vi "RUS Sweep -- write line to log file.vi"(6 "temperature boxes":T1={"LTC21 Address"="GPIB0::15::INSTR", "ITC503 Address"="GPIB0::24::INSTR", "ITC temperature"=299.2, "ITC set temperature"=295.0, "LTC temperature"=0.0, "heater"=0.0, "gas flow"=90.0, "P"=10.0, "D"=1.0, "I"=3.0, "ITC state"="X0A1C2S00H1L0\r", "nonzero temperature"=0.0, "Magn Field (T)"=0.0, "LakeShore340"="", "LS340 Adress"=0, "Sample Temperature Source"=enum."read T <- LakeShore 340", "Neocera sensor"=1}, 7 "base path":path, 8 "error in (no error)":errorcluster, 9 "current sweep file name":string="Stability_", 10 "base name":string="Stability_", 11 "thermometer snapshot":T3={"ITC Temperature"=0.0, "ITC Set Temperature"=0.0, "LTC Temperature"=0.0, "LTC21 Address"="GPIB0::15::INSTR", "ITC503 Address"="GPIB0::24::INSTR"}) -> (0 "error out":errorcluster={"status"=TRUE, "code"=-200019, "source"="DAQmx Read (Analog 1D Wfm NChan NSamp).vi:1<append>\n<B>Task Name: </B>_unnamedTask<2C36>"}, 2 "writing to":string, 3 "log line":string="time=Jun11,2011__19:39:45\tLTC=141.78200\tITC=142.45000\t ITC_set=142.45000\t\t filename=141.78200K_300_3300_061111.dat\t")   [LabVIEW 2015]
uses:
  state.ctl
  Sample_Temperature_Source_Control.ctl
  <vilib>/Utility/file.llb/Write To Spreadsheet File (string).vi
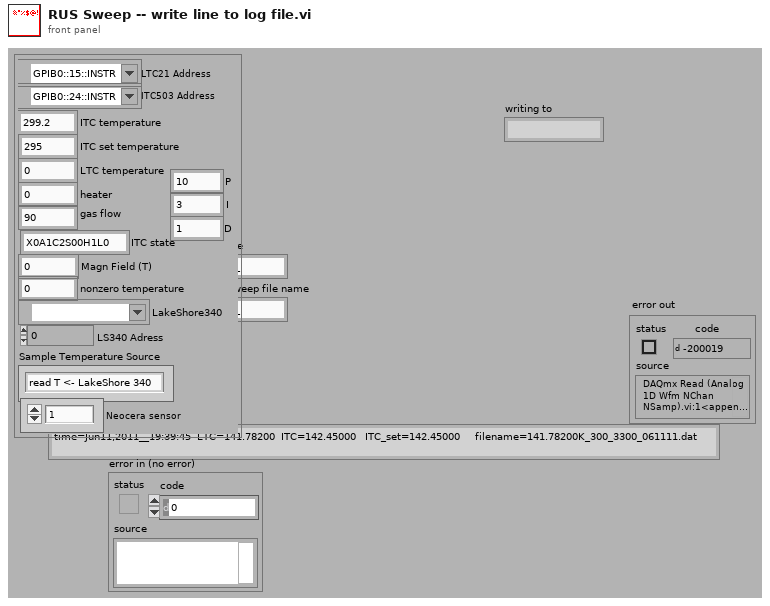
[diagram p1: front panel]
types:
  T1 = typedef "state.ctl" = cluster{"LTC21 Address":refnum<visa-resource-name>, "ITC503 Address":refnum<visa-resource-name>, "ITC temperature":dbl, "ITC set temperature":dbl, "LTC temperature":dbl, "heater":dbl, "gas flow":dbl, "P":dbl, "D":dbl, "I":dbl, "ITC state":string, "nonzero temperature":dbl, "Magn Field (T)":dbl, "LakeShore340":refnum<visa-resource-name>, "LS340 Adress":i16, "Sample Temperature Source":T2, "Neocera sensor":i32}
  T2 = typedef "Sample_Temperature_Source_Control.ctl" = enum16{"read T <- LakeShore 340", "read T <- Neocera"}
  T3 = cluster{"ITC Temperature":dbl, "ITC Set Temperature":dbl, "LTC Temperature":dbl, "LTC21 Address":refnum<visa-resource-name>, "ITC503 Address":refnum<visa-resource-name>}
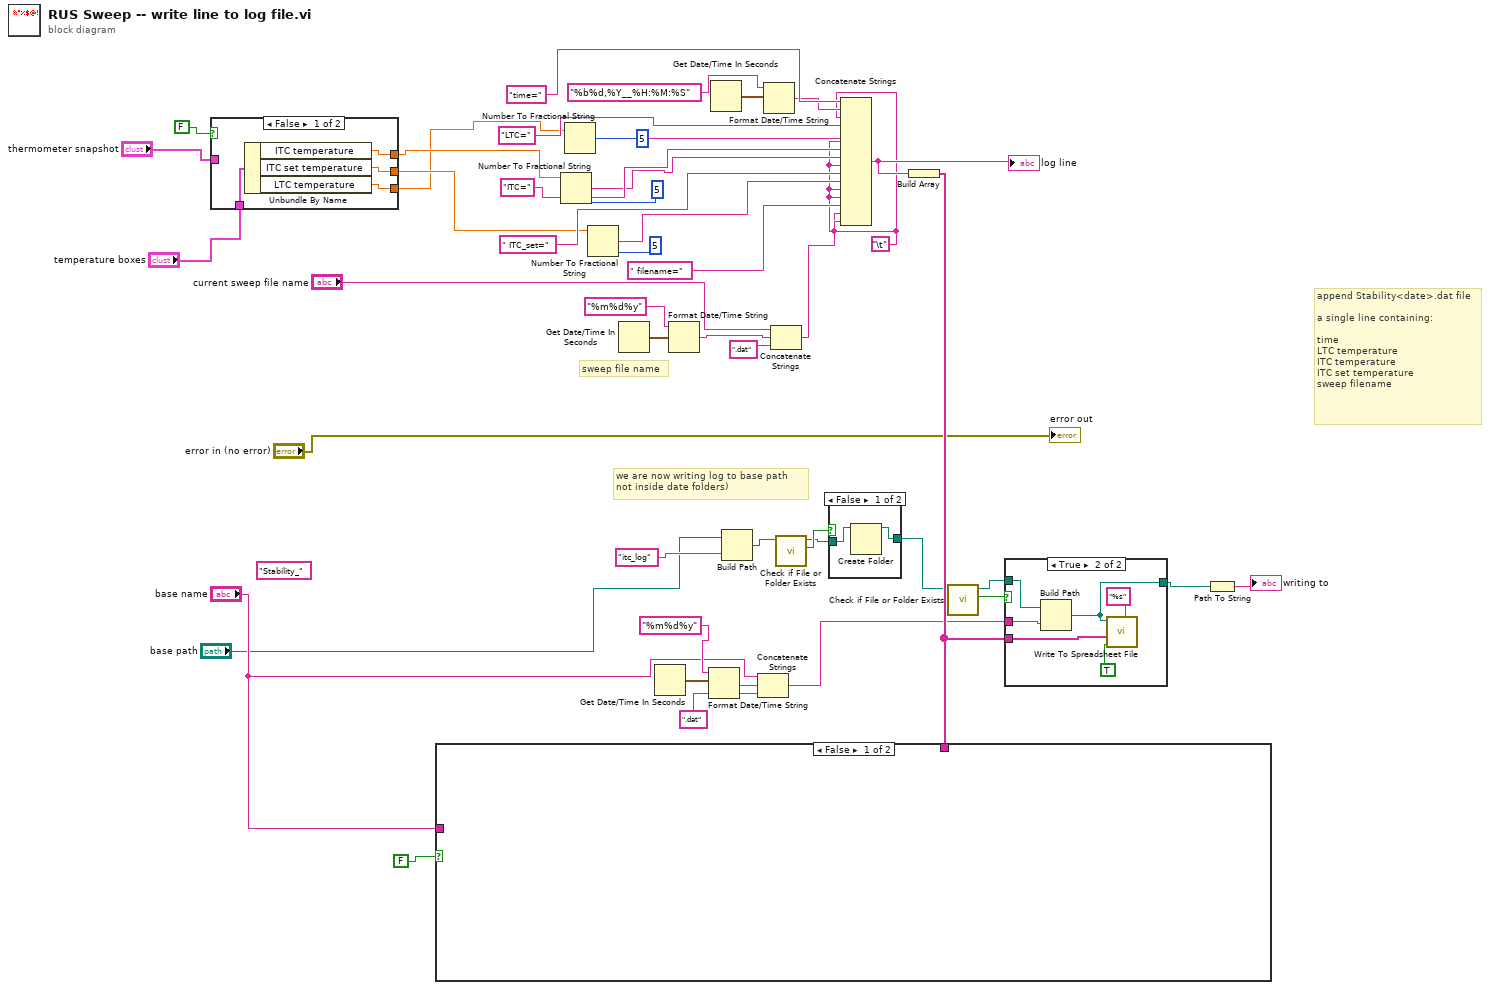
[diagram p0: block diagram]
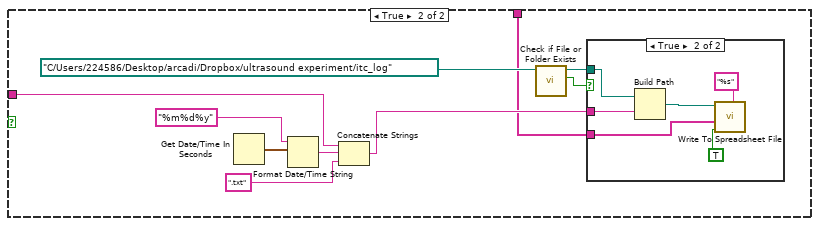
[diagram p2: hidden frame]
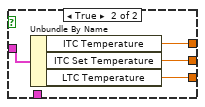
[diagram p5: hidden frame]
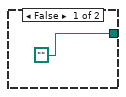
[diagram p6: hidden frame]
diagram:
  w28 = "\t"
  (unwired) "Stability_" ("string")
  # "we are now writing log to base path \nnot inside date folders)"
  # "sweep file name"
  # "append Stability<date>.dat file\n\na single line containing:\n\ntime \nLTC temperature\nITC temperature\nITC set temperature\nsweep filename"
  n1 = case shown="False" FALSE {
    tunnel: "thermometer snapshot" -> [_ w55]
    tunnel: [w51 w54] -> w10
    tunnel: [w50 w53] -> w9
    tunnel: [w49 w52] -> w8
    tunnel: "temperature boxes" -> [w48 _]
    frame False {
      n2 = Unbundle By Name(w48) -> ("ITC temperature"=w51:dbl, "ITC set temperature"=w50:dbl, "LTC temperature"=w49:dbl)
    }
    frame True {
      n3 = Unbundle By Name(w55) -> ("ITC Temperature"=w54:dbl, "ITC Set Temperature"=w53:dbl, "LTC Temperature"=w52:dbl)
    }
  }
  n4 = Number To Fractional String(number=w10, precision (6)=i16 5 ("width (-)")) -> (F-format string=w34:string)  [unwired: 2 in]
  n5 = Number To Fractional String(number=w8, precision (6)=i16 5 ("width (-)")) -> (F-format string=w36:string)  [unwired: 2 in]
  n6 = Number To Fractional String(number=w9, precision (6)=i16 5 ("width (-)")) -> (F-format string=w32:string)  [unwired: 2 in]
  n7 = Get Date/Time In Seconds() -> (seconds since 1Jan1904=w27:timestamp)
  n8 = Get Date/Time In Seconds() -> (seconds since 1Jan1904=w47:timestamp)
  n9 = Format Date/Time String(time format string (%c)="%m%d%y", seconds (now)=w27) -> (date/time string=w26:string)  [unwired: 1 in]
  n10 = Format Date/Time String(time format string (%c)="%m%d%y", seconds (now)=w47) -> (date/time string=w45:string)  [unwired: 1 in]
  n11 = Get Date/Time In Seconds() -> (seconds since 1Jan1904=w43:timestamp)
  n12 = Build Path(base path="base path", name or relative path="itc_log" ("time format string (%c)")) -> (appended path=w6:path)
  n13 = Concatenate Strings("base name", w45, ".dat" ("string")) -> (w15:string)
  n14 = Format Date/Time String(time format string (%c)="%b%d,%Y__%H:%M:%S", seconds (now)=w43) -> (date/time string=w41:string)  [unwired: 1 in]
  n15 = Concatenate Strings("current sweep file name", w26, ".dat" ("string")) -> (w23:string)
  n16 = call <vilib>:"Check if File or Folder Exists.vi"("path"=w6) -> ("file or folder exists?"=w5:bool, "dup path"=w3:path)  [unwired: 8 in, 1 out]
  n17 = case shown="False" w5 {
    tunnel: [w56 w58] -> w2
    tunnel: w3 -> [w57 w58]
    frame False {
      n18 = Create Folder(path (use dialog)=w57) -> (created path=w56:path)  [unwired: 2 in, 2 out]
    }
    frame True {
    }
  }
  n19 = Concatenate Strings("time=" ("string"), w41, w28, "LTC=" ("string"), w36, w28, "ITC=" ("string"), w34, w28, " ITC_set=" ("string"), w32, w28, w28, " filename=" ("string"), w23, w28) -> (w30:string)
  "log line" <- w30
  n20 = Build Array(w30) -> (w18:string[])
  n21 = case shown="False" FALSE {
    tunnel: "base name" -> [_ w63]
    tunnel: w18 -> [_ w60]
    frame False {
    }
    frame True {
      n22 = Get Date/Time In Seconds() -> (seconds since 1Jan1904=w66:timestamp)
      n23 = Format Date/Time String(time format string (%c)="%m%d%y", seconds (now)=w66) -> (date/time string=w65:string)  [unwired: 1 in]
      n24 = Concatenate Strings(w63, w65, ".txt" ("string")) -> (w62:string)
      n25 = call <vilib>:"Check if File or Folder Exists.vi"("path"=path "C:/Users/224586/Desktop/arcadi/Dropbox/ultrasound experiment/itc_log") -> ("file or folder exists?"=w67:bool, "dup path"=w59:path)  [unwired: 8 in, 1 out]
      n26 = case shown="True" w67 {
        tunnel: w59 -> [_ w71]
        tunnel: w62 -> [_ w70]
        tunnel: w60 -> [_ w69]
        frame False {
        }
        frame True {
          n27 = Build Path(base path=w71, name or relative path=w70) -> (appended path=w72:path)
          n28 = call-poly <vilib>:"Write To Spreadsheet File.vi"("format (%s)"="%s", "append to file? (new file:F)"=TRUE, "1D data"=w69, "file path (dialog if empty)"=w72) -> ()  [unwired: 4 in, 1 out]
        }
      }
    }
  }
  n29 = call <vilib>:"Check if File or Folder Exists.vi"("path"=w2) -> ("file or folder exists?"=w20:bool, "dup path"=w16:path)  [unwired: 8 in, 1 out]
  n30 = case shown="True" w20 {
    tunnel: w18 -> [_ w79]
    tunnel: w16 -> [_ w78]
    tunnel: w15 -> [_ w77]
    tunnel: [path "" w76] -> w14
    frame False {
    }
    frame True {
      n31 = Build Path(base path=w78, name or relative path=w77) -> (appended path=w76:path)
      n32 = call-poly <vilib>:"Write To Spreadsheet File.vi"("format (%s)"="%s", "append to file? (new file:F)"=TRUE, "1D data"=w79, "file path (dialog if empty)"=w76) -> ()  [unwired: 4 in, 1 out]
    }
  }
  n33 = Path To String(path=w14) -> (string=→"writing to":string)
  "error out" <- "error in (no error)"
